vi "solar_voy HS DB.vi"(0 "HDR_GUID":string, 2 "Action":enum8{"DELETE", "ADD", "CLEAR"}(ring), 5 "ORIGIN in":enum8{"RMT", "LCL"}(ring), 7 "TARGET in":string, 9 "PACKET in":string, 11 "DATA in":string) -> (4 "Exists?":bool, 6 "ORIGIN out":enum8{"RMT", "LCL"}(ring), 8 "TARGET out":string, 10 "PACKET out":string, 15 "DATA out":string)   [LabVIEW 2018]
doc: "This functional global records the 'HDR_GUID' and original message to be used when the 'HANDSHAKE' message is returned."
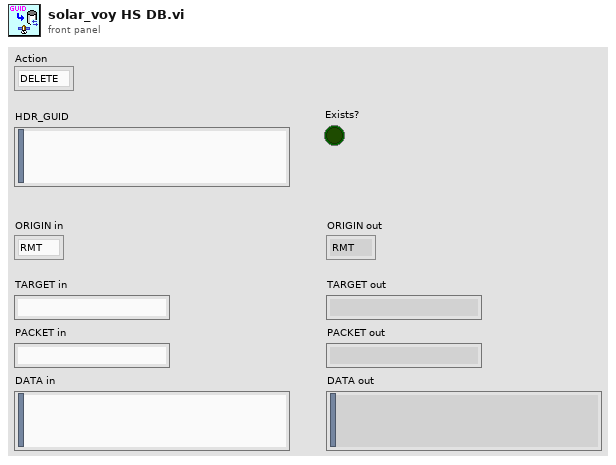
[diagram p1: front panel]
types:
  T1 = cluster{"HDR_GUID":string, "ORIGIN":enum8{"RMT", "LCL"}, "TARGET":string, "PACKET":string, "DATA":string}
  T2 = cluster{"HDR_GUID":string, "ORIGIN":enum8{"RMT", "LCL"}, "TARGET":string, "PACKET":string, "DATA":string}[]
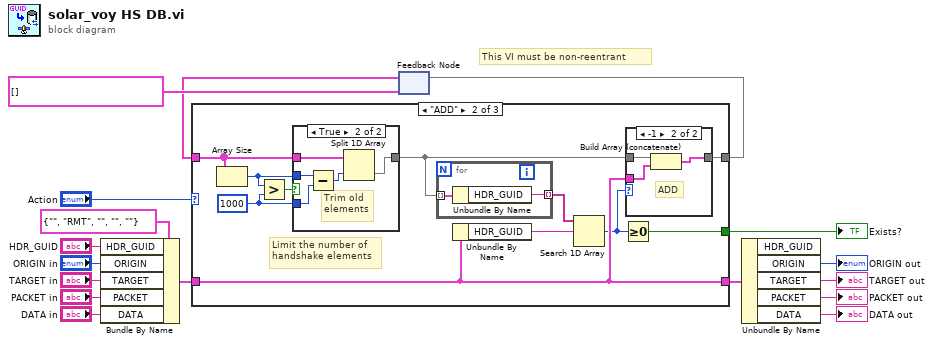
[diagram p0: block diagram]
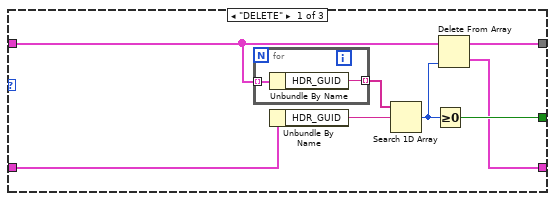
[diagram p2: hidden frame]
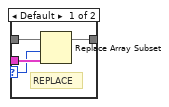
[diagram p4: hidden frame]
diagram:
  # "This VI must be non-reentrant"
  n1 = Bundle By Name(cluster=T1 {"HDR_GUID"="", "ORIGIN"=enum."RMT", "TARGET"="", "PACKET"="", "DATA"=""} ("GUID"), "HDR_GUID"="HDR_GUID", "ORIGIN"="ORIGIN in", "TARGET"="TARGET in", "PACKET"="PACKET in", "DATA"="DATA in") -> (w15:T1)
  n2 = feedback #1(T2 [] ("GUID")) -> (w3:T2)
  n3 = case shown="\"ADD\"" "Action" {
    tunnel: [w24 w33 _] -> w16
    tunnel: w15 -> [w22 w35 _]
    tunnel: [w20 w35 _] -> w13
    tunnel: w3 -> [w19 w32 _]
    tunnel: [w18 w36 _] -> w1
    frame "DELETE" {
      n4 = for {
        tunnel: w19 -> [w27] mode=indexing
        tunnel: [w26] -> w25 mode=indexing
        n5 = Unbundle By Name(w27) -> ("HDR_GUID"=w26:string)
      }
      n6 = Unbundle By Name(w22) -> ("HDR_GUID"=w21:string)
      n7 = Search 1D Array(1D array=w25, element=w21) -> (index of element=w23:i32)  [unwired: 1 in]
      n8 = Greater Or Equal To 0?(x=w23) -> (x >= 0?=w24:bool)
      n9 = Delete From Array(array=w19, index=w23) -> (deleted portion=w20:T1, array with subset deleted=w18:T2)  [unwired: 1 in]
    }
    frame "ADD" {
      w29 = 1000 ("y")
      # "Limit the number of\nhandshake elements"
      n10 = Array Size(array=w32) -> (size(s)=w30:i32)
      n11 = Greater?(x=w30, y=w29) -> (0:w31:bool)
      n12 = case shown="True" w31 {
        tunnel: w32 -> [w39 w44]
        tunnel: [w39 w43] -> w28
        tunnel: w30 -> [_ w42]
        tunnel: w29 -> [_ w41]
        frame False {
          # "Less than\nlimit"
        }
        frame True {
          # "Trim old\nelements"
          n13 = Subtract(x=w42, y=w41) -> (x-y=w40:i32)
          n14 = Split 1D Array(array=w44, index=w40) -> (second subarray=w43:T2)  [unwired: 1 out]
        }
      }
      n15 = for {
        tunnel: w28 -> [w53] mode=indexing
        tunnel: [w52] -> w38 mode=indexing
        n16 = Unbundle By Name(w53) -> ("HDR_GUID"=w52:string)
      }
      n17 = Unbundle By Name(w35) -> ("HDR_GUID"=w37:string)
      n18 = Search 1D Array(1D array=w38, element=w37) -> (index of element=w34:i32)  [unwired: 1 in]
      n19 = Greater Or Equal To 0?(x=w34) -> (x >= 0?=w33:bool)
      n20 = case shown="-1" w34 {
        selector: w34 -> [w45 _]
        tunnel: [w47 w50] -> w36
        tunnel: w28 -> [w48 w51]
        tunnel: w35 -> [w46 w49]
        frame Default {
          # "REPLACE"
          n21 = Replace Array Subset(array=w48, new element=w46, index=w45) -> (w47:T2)
        }
        frame -1 {
          # "ADD"
          n22 = Build Array (concatenate)(w51, w49) -> (w50:T2)
        }
      }
    }
    frame "CLEAR" {
    }
  }
  "Exists?" <- w16
  n23 = feedback-in #1(w1) -> ()
  n24 = Unbundle By Name(w13) -> ("ORIGIN"=→"ORIGIN out":enum8{"RMT", "LCL"}, "TARGET"=→"TARGET out":string, "PACKET"=→"PACKET out":string, "DATA"=→"DATA out":string)  [unwired: 1 out]
